vi "Start IO Tasks.vi"(8 "error in (no error)":errorcluster, 11 "BaseProducer in":refnum<class "BaseProducer.lvclass">) -> (0 "error out":errorcluster, 3 "BaseProducer out":refnum<class "BaseProducer.lvclass">)   [LabVIEW 2013, in "BaseProducer.lvclass"]
doc: "This method starts IO tasks for the current experiment, determines the clock rate for the dynamic pressure sensors, and turns out remote enable digital outputs for controlling the MFCs."
uses:
  BaseProducer.lvclass
  BaseProducer.lvclass/BaseProducer.ctl
  <vilib>/DAQmx/write.llb/DAQmx Write (Digital 1D Bool NChan 1Samp 1Line).vi
  <vilib>/DAQmx/miscellaneous.llb/DAQmx Fill In Error Info.vi
  <resource>/objmgr/daqmx.rc
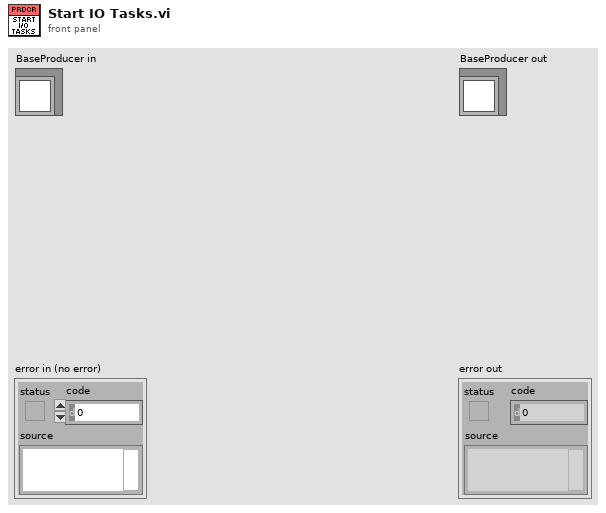
[diagram p1: front panel]
types:
  T1 = typedef "BaseProducer.lvclass/IO Task Cluster.ctl" = cluster{"Dynamic P Tasks":refnum<k21>, "AI Tasks":refnum<k21>, "DIO Tasks":refnum<k21>, "AO Tasks":refnum<k21>}
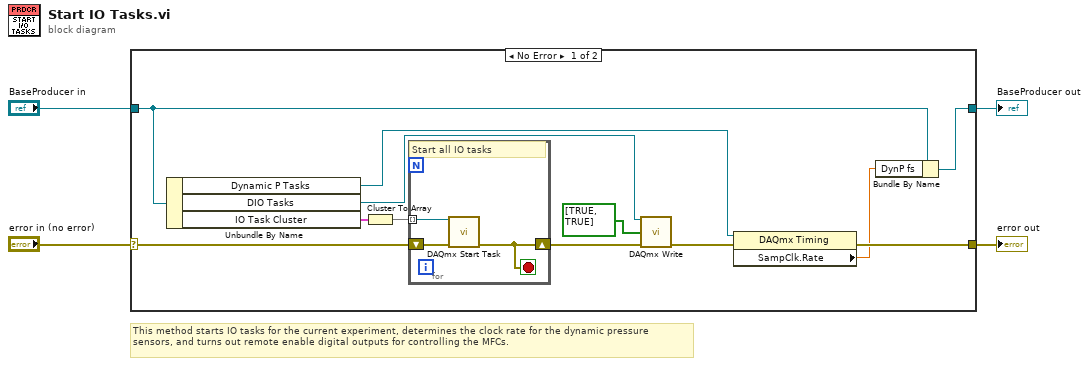
[diagram p0: block diagram]
diagram:
  # "This method starts IO tasks for the current experiment, determines the clock rate for the dynamic pressure sensors, and turns out remote enable digital outputs for controlling the MFCs."
  n1 = case shown="No Error" "error in (no error)" {
    selector: "error in (no error)" -> [w16 w21]
    tunnel: [w8 w21] -> w3
    tunnel: [w6 w20] -> w1
    tunnel: "BaseProducer in" -> [w7 w20]
    frame No Error {
      n2 = Unbundle By Name(w7) -> ("Dynamic P Tasks"=w9:refnum<k21>, "DIO Tasks"=w12:refnum<k21>, "IO Task Cluster"=w15:T1)
      n3 = Cluster To Array(cluster=w15) -> (array=w14:refnum<k21>[])
      n4 = for {
        shift-right: [w18] -> w13
        shift-left: w16 -> [w19]
        tunnel: w14 -> [w17] mode=indexing
        stop <- w18 stop-if-true
        # "Start all IO tasks"
        n5 = call <vilib>:"DAQmx Start Task.vi"("task/channels in"=w17, "error in"=w19) -> ("error out"=w18:errorcluster)  [unwired: 12 in, 1 out]
      }
      n6 = call-poly <vilib>:"DAQmx Write.vi"("task/channels in"=w12, "data"=bool[] [TRUE, TRUE], "error in"=w13) -> ("error out"=w10:errorcluster)  [unwired: 10 in, 2 out]
      n7 = property class="DAQmx Timing"(reference=w9, error in=w10) -> (error out=w8:errorcluster, "SampClk.Rate"=w5:dbl)  [unwired: 1 out]
      n8 = Bundle By Name(cluster=w7, "DynP fs"=w5) -> (w6:refnum<class "BaseProducer.lvclass">)
    }
    frame Error {
    }
  }
  "error out" <- w3
  "BaseProducer out" <- w1
